vi "Measurement.Init.vi"(8 "error in (no error)":errorcluster, 10 "timeout (5000 ms)":i32=5000, 11 "Measurement.WavelengthSweeping in":refnum<class "Measurement.WavelengthSweeping.lvclass">) -> (0 "error out":errorcluster, 1 "Dependencies Results":bool[](array[boolean]), 2 "Result":bool, 3 "Measurement.WavelengthSweeping out":refnum<class "Measurement.WavelengthSweeping.lvclass">)   [LabVIEW 2017, in "Measurement.WavelengthSweeping.lvclass"]
uses:
  Measurement.WavelengthSweeping.lvclass
  MC/MC/MC.lvclass
  D:/upwork/Laser Measurement Tool/Laser/project/Subsystems/Device/Device.lvclass
  SMU/SMU.lvclass
  OPA/OPA.lvclass
  OPM/OPM.lvclass
  LIA/LIA.lvclass
  Device/Device.lvclass
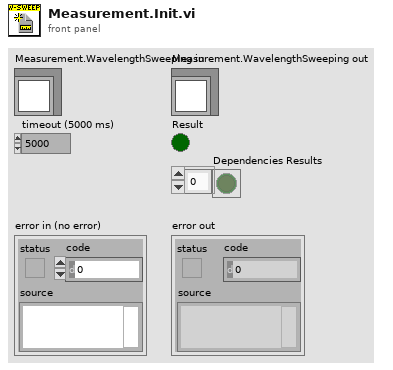
[diagram p1: front panel]
types:
  T1 = typedef "Measurement.WavelengthSweeping.lvclass/Configuration--Cluster.ctl" = cluster{"Measurement.Type":T2, "Hardware":T3, "Measurement":T14}
  T2 = typedef "Measurement.lvclass/Measurement.Type--Enum.ctl" = enum16{"Free", "I/V Curve", "Wavelength sweeping", "Photocurrent mapping"}
  T3 = typedef "Measurement.WavelengthSweeping.lvclass/Configuration.Hardware--Cluster.ctl" = cluster{"SMU":T4, "LIA":T6, "OPM":T8, "OPA":T10, "MC":T12}
  T4 = typedef "Measurement.lvclass/Configuration.SMU--Cluster.ctl" = cluster{"Enable":bool, "SMU Model":string, "Configuration":T5}
  T5 = typedef "SMU.lvclass/Configuration--Cluster.ctl" = cluster{"VISA Resource":string, "Channel":string}
  T6 = typedef "Measurement.lvclass/Configuration.LIA--Cluster.ctl" = cluster{"Enable":bool, "LIA Model":string, "Configuration":T7}
  T7 = typedef "LIA.lvclass/Configuration--Cluster.ctl" = cluster{"VISA Resource":string}
  T8 = typedef "Measurement.lvclass/Configuration.OPM--Cluster.ctl" = cluster{"Enable":bool, "OPM Model":string, "Configuration":T9}
  T9 = typedef "OPM.lvclass/Configuration--Cluster.ctl" = cluster{"VISA Resource":string}
  T10 = typedef "Measurement.lvclass/Configuration.OPA--Cluster.ctl" = cluster{"Enable":bool, "OPA Model":string, "Configuration":T11}
  T11 = typedef "OPA.lvclass/Configuration--Cluster.ctl" = cluster{"Serial Number":string}
  T12 = typedef "Measurement.lvclass/Configuration.MC--Cluster.ctl" = cluster{"Enable":bool, "MC Model":string, "Configuration":T13}
  T13 = typedef "MC.lvclass/Configuration--Cluster.ctl" = cluster{"VISA Resource":string}
  T14 = typedef "Measurement.WavelengthSweeping.lvclass/Configuration.Measurement--Cluster.ctl" = cluster{"SMU Voltage, V":dbl, "OPA Start wavelength, nm":dbl, "OPA Stop wavelength, nm":dbl, "OPA Scan resolution, nm":dbl, "OPA Number or points":u16, "Integration time, sec":dbl, "Delay time, ms":u16, "Accumulation":u16}
  T15 = typedef "Measurement.WavelengthSweeping.lvclass/Dependencies--Cluster.ctl" = cluster{"SMU":refnum<class "SMU.lvclass">, "LIA":refnum<class "LIA.lvclass">, "OPM":refnum<class "OPM.lvclass">, "OPA":refnum<class "OPA.lvclass">, "MC":refnum<class "MC.lvclass">}
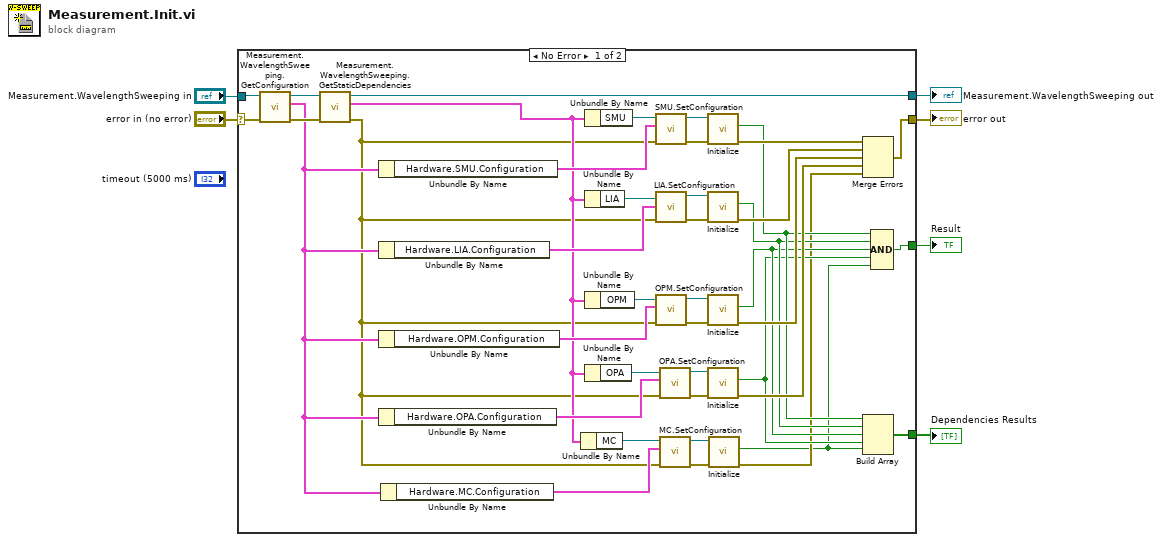
[diagram p0: block diagram]
diagram:
  n1 = case shown="No Error" "error in (no error)" {
    selector: "error in (no error)" -> [w46 w48]
    tunnel: "Measurement.WavelengthSweeping in" -> [w47 w49]
    tunnel: [w19 w49] -> w4
    tunnel: [w18 w48] -> w3
    tunnel: [w17 _] -> w1
    tunnel: [w16 _] -> w2
    frame No Error {
      n2 = call "Measurement.WavelengthSweeping.GetConfiguration.vi"("error in (no error)"=w46, "Measurement.WavelengthSweeping"=w47) -> ("error out"=w44:errorcluster, "Configuration"=w13:T1, "Measurement.WavelengthSweeping out"=w45:refnum<class "Measurement.WavelengthSweeping.lvclass">)  [unwired: 7 in]
      n3 = call "Measurement.WavelengthSweeping.GetStaticDependencies.vi"("error in (no error)"=w44, "Measurement.WavelengthSweeping in"=w45) -> ("error out"=w11:errorcluster, "Dependencies"=w12:T15, "Measurement.WavelengthSweeping out"=w19:refnum<class "Measurement.WavelengthSweeping.lvclass">)  [unwired: 7 in]
      n4 = Unbundle By Name(w13) -> ("Hardware.SMU.Configuration"=w42:T5)
      n5 = Unbundle By Name(w13) -> ("Hardware.LIA.Configuration"=w37:T7)
      n6 = Unbundle By Name(w13) -> ("Hardware.OPM.Configuration"=w32:T9)
      n7 = Unbundle By Name(w13) -> ("Hardware.OPA.Configuration"=w27:T11)
      n8 = Unbundle By Name(w13) -> ("Hardware.MC.Configuration"=w14:T13)
      n9 = Unbundle By Name(w12) -> ("MC"=w15:refnum<class "MC.lvclass">)
      n10 = Unbundle By Name(w12) -> ("SMU"=w43:refnum<class "SMU.lvclass">)
      n11 = Unbundle By Name(w12) -> ("LIA"=w38:refnum<class "LIA.lvclass">)
      n12 = Unbundle By Name(w12) -> ("OPM"=w33:refnum<class "OPM.lvclass">)
      n13 = Unbundle By Name(w12) -> ("OPA"=w28:refnum<class "OPA.lvclass">)
      n14 = call "SMU.SetConfiguration.vi"("error in (no error)"=w11, "Configuration"=w42, "SMU"=w43) -> ("error out"=w40:errorcluster, "SMU out"=w41:refnum<class "SMU.lvclass">)  [unwired: 7 in]
      n15 = call "LIA.SetConfiguration.vi"("error in (no error)"=w11, "Configuration"=w37, "LIA"=w38) -> ("error out"=w36:errorcluster, "LIA out"=w35:refnum<class "LIA.lvclass">)  [unwired: 7 in]
      n16 = call "OPM.SetConfiguration.vi"("error in (no error)"=w11, "Configuration"=w32, "PM"=w33) -> ("error out"=w30:errorcluster, "PM out"=w31:refnum<class "OPM.lvclass">)  [unwired: 7 in]
      n17 = call "OPA.SetConfiguration.vi"("error in (no error)"=w11, "Configuration"=w27, "OPA"=w28) -> ("error out"=w26:errorcluster, "OPA out"=w25:refnum<class "OPA.lvclass">)  [unwired: 7 in]
      n18 = call "MC.SetConfiguration.vi"("error in (no error)"=w11, "Configuration"=w14, "MC"=w15) -> ("error out"=w10:errorcluster, "MC out"=w9:refnum<class "MC.lvclass">)  [unwired: 7 in]
      n19 = call "Initialize.vi"("error in (no error)"=w40, "Device in"=w41) -> ("error out"=w39:errorcluster, "Result"=w23:bool)  [unwired: 7 in, 1 out]
      n20 = call "Initialize.vi"("error in (no error)"=w36, "Device in"=w35) -> ("error out"=w34:errorcluster, "Result"=w22:bool)  [unwired: 7 in, 1 out]
      n21 = call "Initialize.vi"("error in (no error)"=w30, "Device in"=w31) -> ("error out"=w29:errorcluster, "Result"=w21:bool)  [unwired: 7 in, 1 out]
      n22 = call "Initialize.vi"("error in (no error)"=w26, "Device in"=w25) -> ("error out"=w24:errorcluster, "Result"=w20:bool)  [unwired: 7 in, 1 out]
      n23 = call "Initialize.vi"("error in (no error)"=w10, "Device in"=w9) -> ("error out"=w8:errorcluster, "Result"=w7:bool)  [unwired: 7 in, 1 out]
      n24 = Merge Errors(w39, w34, w29, w24, w8) -> (w18:errorcluster)
      n25 = Build Array(w23, w22, w21, w20, w7) -> (w16:bool[])
      n26 = Compound Arithmetic op=AND(w23, w22, w21, w20, w7) -> (w17:bool)
    }
    frame Error {
    }
  }
  "error out" <- w3
  "Measurement.WavelengthSweeping out" <- w4
  "Result" <- w1
  "Dependencies Results" <- w2
